vi "Get Reference.vi"(8 "error in (no error)":errorcluster, 10 "Samples":i32, 11 "Software Lock-in in":refnum<class "Software Lock-in.lvclass">) -> (0 "error out":errorcluster, 2 "Reference":cdb[](array[numeric]), 3 "Software Lock-in out":refnum<class "Software Lock-in.lvclass">)   [LabVIEW 2015, in "Software Lock-in.lvclass"]
uses:
  Software Lock-in.lvclass
  Software Lock-in.lvclass/Software Lock-in.ctl
  <vilib>/Analysis/NI_AALBase.lvlib
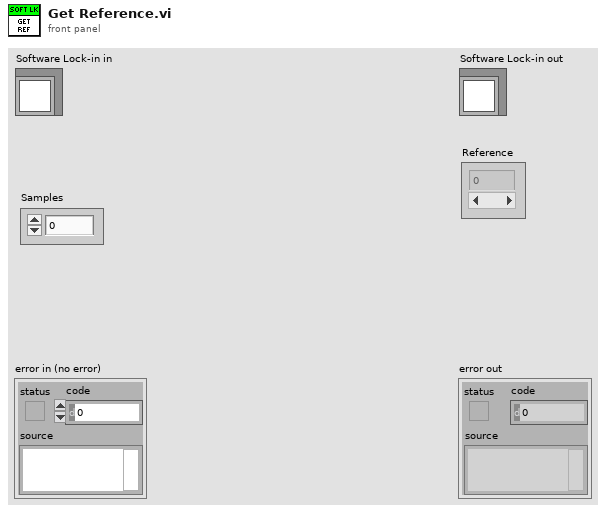
[diagram p1: front panel]
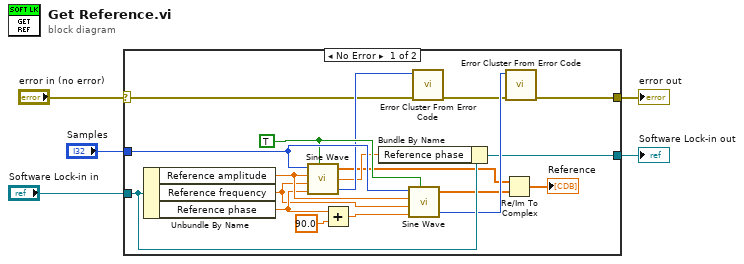
[diagram p0: block diagram]
diagram:
  n1 = case shown="No Error" "error in (no error)" {
    selector: "error in (no error)" -> [w15 w25]
    tunnel: [w13 w25] -> w4
    tunnel: [w11 w24] -> w2
    tunnel: "Software Lock-in in" -> [w20 w24]
    tunnel: "Samples" -> [w21 _]
    frame No Error {
      w18 = TRUE ("reset phase")
      n2 = Unbundle By Name(w20) -> ("Reference amplitude"=w19:dbl, "Reference frequency"=w9:dbl, "Reference phase"=w12:dbl)
      n3 = call <vilib>:"Sine Wave.vi"("samples"=w21, "amplitude"=w19, "frequency"=w9, "phase in"=w12, "reset phase"=w18) -> ("sine wave"=w8:dbl[], "phase out"=w10:dbl, "error"=w17:i32)
      n4 = Add(x=w12, y=90.0) -> (x+y=w22:dbl)
      n5 = Bundle By Name(cluster=w20, "Reference phase"=w10) -> (w11:refnum<class "Software Lock-in.lvclass">)
      n6 = call <vilib>:"Sine Wave.vi"("samples"=w21, "amplitude"=w19, "frequency"=w9, "phase in"=w22, "reset phase"=w18) -> ("sine wave"=w7:dbl[], "error"=w16:i32)  [unwired: 1 out]
      n7 = call <vilib>:"Error Cluster From Error Code.vi"("error in (no error)"=w15, "error code (0)"=w17) -> ("error out"=w14:errorcluster)  [unwired: 7 in]
      n8 = Re/Im To Complex(1:w7, 2:w8) -> (0:→"Reference":cdb[])
      n9 = call <vilib>:"Error Cluster From Error Code.vi"("error in (no error)"=w14, "error code (0)"=w16) -> ("error out"=w13:errorcluster)  [unwired: 7 in]
    }
    frame Error {
    }
  }
  "error out" <- w4
  "Software Lock-in out" <- w2
